vi "Outputs.vi"(8 "error in (no error)":errorcluster, 11 "State in":T1={"State"=enum."Idle", "Start Time"=timestamp(0 s since 1904-01-01), "Configuration"={"Cycle Period"=0.0, "Ismatech"={"VISA resource name"="", "Simulated?"=FALSE, "Pump Number"=1.0, "Reverse?"=FALSE}, "Masterflex"={"VISA resource name"="", "Simulated?"=FALSE, "Pump Number"=1.0, "Reverse?"=FALSE}, "Mettler"={"VISA resource name"="", "Simulated?"=FALSE}, "Bronkhorst M13 Flow Meter"={"VISA resource name"="", "Simulated?"=FALSE, "Smoothing Steps"=1}, "PID 2 Parameters"={"Input Device"=enum."Flowmeter", "Output Device"=enum."Ismatec ISM 831C", "Setpoint"=0.0, "PID gains"={"proportional gain (Kc)"=1.0, "integral time (Ti, min)"=0.01, "derivative time (Td, min)"=0.0}}, "Manual Entry"=0.0, "Auto?"=TRUE, "VICI Settings"={"VISA resource name"="", "Simulated?"=FALSE, "Pump Number"=0.0, "Reverse?"=FALSE}, "output range"={"output high"=100.0, "output low"=0.0}}, "Current Time"=timestamp(0 s since 1904-01-01), "PID 1 Parameters"={"Setpoint"=0.0, "PID gains"={"proportional gain (Kc)"=1.0, "integral time (Ti, min)"=0.01, "derivative time (Td, min)"=0.0}}, "First Iteration"=FALSE, "Data"={"Flowmeter Output"=0.0, "PID 1 Output"=0.0, "PID 2 Process Variable"=0.0, "Scale Output (g)"=0.0, "PID 2 output"=0.0, "Scale Rate of Change (g/min)"=0.0}, "Process Name"="", "Pump On?"=FALSE} {"PID 1 Parameters"."PID gains"."derivative time (Td, min)" format="%.3f"; "PID 1 Parameters"."PID gains"."integral time (Ti, min)" format="%.3f"; "PID 1 Parameters"."PID gains"."proportional gain (Kc)" format="%.3f"; "Configuration"."output range"."output low" min=0.0 max=100.0 format="%.2f"; "Configuration"."output range"."output high" format="%.2f"; "Configuration"."VICI Settings"."Pump Number" min=1.0 max=20.0 step=1.0; "Configuration"."PID 2 Parameters"."PID gains"."derivative time (Td, min)" format="%.3f"; "Configuration"."PID 2 Parameters"."PID gains"."integral time (Ti, min)" format="%.3f"; "Configuration"."PID 2 Parameters"."PID gains"."proportional gain (Kc)" format="%.3f"; "Configuration"."Bronkhorst M13 Flow Meter"."Smoothing Steps" min=1 step=1; "Configuration"."Masterflex"."Pump Number" min=1.0 max=20.0 step=1.0; "Configuration"."Ismatech"."Pump Number" min=1.0 max=20.0 step=1.0}) -> (0 "error out":errorcluster, 3 "State out":T1={"State"=enum."Idle", "Start Time"=timestamp(0 s since 1904-01-01), "Configuration"={"Cycle Period"=0.0, "Ismatech"={"VISA resource name"="", "Simulated?"=FALSE, "Pump Number"=1.0, "Reverse?"=FALSE}, "Masterflex"={"VISA resource name"="", "Simulated?"=FALSE, "Pump Number"=1.0, "Reverse?"=FALSE}, "Mettler"={"VISA resource name"="", "Simulated?"=FALSE}, "Bronkhorst M13 Flow Meter"={"VISA resource name"="", "Simulated?"=FALSE, "Smoothing Steps"=1}, "PID 2 Parameters"={"Input Device"=enum."Flowmeter", "Output Device"=enum."Ismatec ISM 831C", "Setpoint"=0.0, "PID gains"={"proportional gain (Kc)"=1.0, "integral time (Ti, min)"=0.01, "derivative time (Td, min)"=0.0}}, "Manual Entry"=0.0, "Auto?"=TRUE, "VICI Settings"={"VISA resource name"="", "Simulated?"=FALSE, "Pump Number"=0.0, "Reverse?"=FALSE}, "output range"={"output high"=100.0, "output low"=0.0}}, "Current Time"=timestamp(0 s since 1904-01-01), "PID 1 Parameters"={"Setpoint"=0.0, "PID gains"={"proportional gain (Kc)"=1.0, "integral time (Ti, min)"=0.01, "derivative time (Td, min)"=0.0}}, "First Iteration"=FALSE, "Data"={"Flowmeter Output"=0.0, "PID 1 Output"=0.0, "PID 2 Process Variable"=0.0, "Scale Output (g)"=0.0, "PID 2 output"=0.0, "Scale Rate of Change (g/min)"=0.0}, "Process Name"="", "Pump On?"=FALSE} {"PID 1 Parameters"."PID gains"."derivative time (Td, min)" format="%.3f"; "PID 1 Parameters"."PID gains"."integral time (Ti, min)" format="%.3f"; "PID 1 Parameters"."PID gains"."proportional gain (Kc)" format="%.3f"; "Configuration"."output range"."output low" min=0.0 max=100.0 format="%.2f"; "Configuration"."output range"."output high" format="%.2f"; "Configuration"."VICI Settings"."Pump Number" min=1.0 max=20.0 step=1.0; "Configuration"."PID 2 Parameters"."PID gains"."derivative time (Td, min)" format="%.3f"; "Configuration"."PID 2 Parameters"."PID gains"."integral time (Ti, min)" format="%.3f"; "Configuration"."PID 2 Parameters"."PID gains"."proportional gain (Kc)" format="%.3f"; "Configuration"."Bronkhorst M13 Flow Meter"."Smoothing Steps" min=1 step=1; "Configuration"."Masterflex"."Pump Number" min=1.0 max=20.0 step=1.0; "Configuration"."Ismatech"."Pump Number" min=1.0 max=20.0 step=1.0})   [LabVIEW 2021, in "Scale Module.lvlib" / "Scale Module Engine.lvlib"]
uses:
  Scale Module Engine.lvlib
  Ismatec ISM 831C/Ismatec ISM 831C.lvlib
  Masterflex 7550-30/Masterflex 7550-30.lvlib
  VICI M50/VICI M50.lvlib
  State Enum.ctl
  Feed Module/Controls/Scale Module Settings Cluster.ctl
  Scale Module.lvlib
  State Cluster.ctl
  Measure Instrument/PID Input Enum.ctl
  Measure Instrument/PID 2 Output Enum.ctl
  Measure Instrument/PID 2 Parameters Cluster.ctl
  Ismatec ISM 831C/Controls/Ismatech Settings Cluster.ctl
  Masterflex 7550-30/Controls/Settings Cluster.ctl
  Mettler Toledo/Controls/Settings Cluster.ctl
  Mettler Toledo/Mettler Toledo.lvlib
  Measure Instrument/PID 1 Parameters Cluster.ctl
  VICI M50/VICI Settings.ctl
  Bronkhorst M13 Flow Meter/Settings Cluster.ctl
  Bronkhorst M13 Flow Meter/Bronkhorst M13 Flow Meter.lvlib
panel:
  # "Output Instruments"
  # "Input Instruments"
  # "Output Instruments"
  # "Input Instruments"
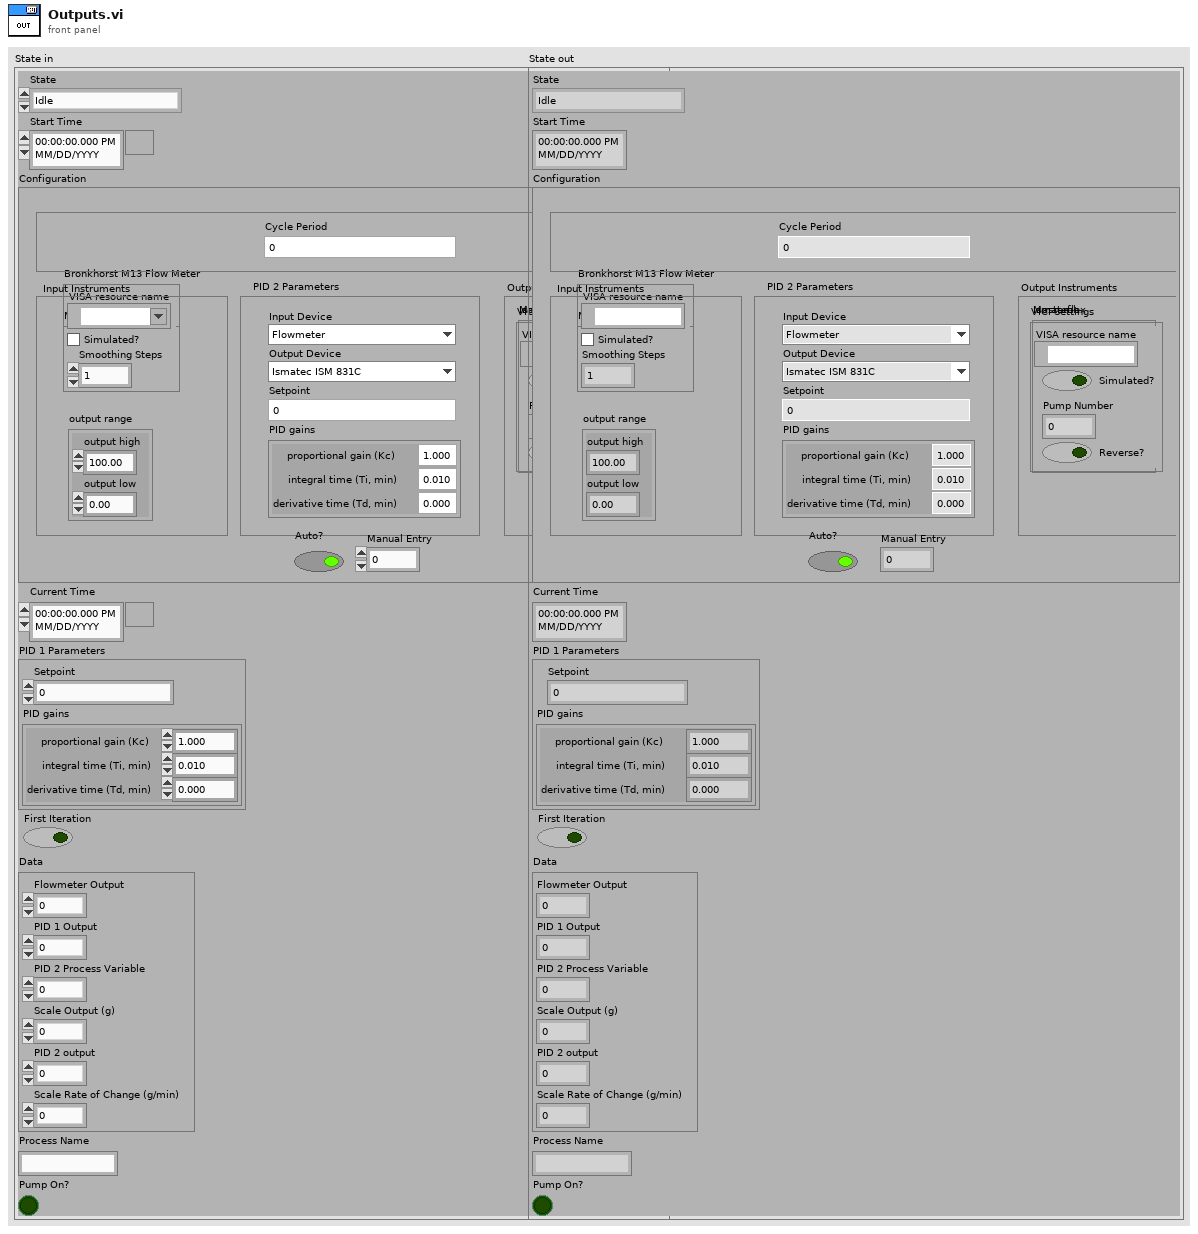
[diagram p1: front panel]
types:
  T1 = typedef "Scale Module.lvlib/Scale Module Engine.lvlib/State Cluster.ctl" = cluster{"State":T2, "Start Time":timestamp, "Configuration":T3, "Current Time":timestamp, "PID 1 Parameters":T12, "First Iteration":bool, "Data":cluster{"Flowmeter Output":dbl, "PID 1 Output":dbl, "PID 2 Process Variable":dbl, "Scale Output (g)":dbl, "PID 2 output":dbl, "Scale Rate of Change (g/min)":dbl}, "Process Name":string, "Pump On?":bool}
  T2 = typedef "Scale Module.lvlib/Scale Module Engine.lvlib/State Enum.ctl" = enum16{"Measuring", "Idle"}
  T3 = typedef "Scale Module.lvlib/Scale Module Settings Cluster.ctl" = cluster{"Cycle Period":dbl, "Ismatech":T4, "Masterflex":T5, "Mettler":T6, "Bronkhorst M13 Flow Meter":T7, "PID 2 Parameters":T8, "Manual Entry":dbl, "Auto?":bool, "VICI Settings":T11, "output range":cluster{"output high":dbl, "output low":dbl}}
  T4 = typedef "Ismatec ISM 831C.lvlib/Ismatech Settings Cluster.ctl" = cluster{"VISA resource name":refnum<visa-resource-name>, "Simulated?":bool, "Pump Number":dbl, "Reverse?":bool}
  T5 = typedef "Masterflex 7550-30.lvlib/Settings Cluster.ctl" = cluster{"VISA resource name":refnum<visa-resource-name>, "Simulated?":bool, "Pump Number":dbl, "Reverse?":bool}
  T6 = typedef "Mettler Toledo.lvlib/Settings Cluster.ctl" = cluster{"VISA resource name":refnum<visa-resource-name>, "Simulated?":bool}
  T7 = typedef "Bronkhorst M13 Flow Meter.lvlib/Settings Cluster.ctl" = cluster{"VISA resource name":refnum<visa-resource-name>, "Simulated?":bool, "Smoothing Steps":i32}
  T8 = typedef "PID 2 Parameters Cluster.ctl" = cluster{"Input Device":T9, "Output Device":T10, "Setpoint":dbl, "PID gains":cluster{"proportional gain (Kc)":dbl, "integral time (Ti, min)":dbl, "derivative time (Td, min)":dbl}}
  T9 = typedef "PID Input Enum.ctl" = enum16{"Default", "Flowmeter", "Scale Rate of Change"}
  T10 = typedef "PID 2 Output Enum.ctl" = enum16{"Default", "Ismatec ISM 4308", "Ismatec ISM 831C", "Masterflex 7550-30", "VICI M6", "VICI M50", "Tacmina QI", "KNF SIMDOS", "ASIA Type C", "FLOM UI-22-11", "SSI PR/LD", "SSI P40", "Masterflex 75211-70"}
  T11 = typedef "VICI Settings.ctl" = cluster{"VISA resource name":refnum<visa-resource-name>, "Simulated?":bool, "Pump Number":dbl, "Reverse?":bool}
  T12 = typedef "PID 1 Parameters Cluster.ctl" = cluster{"Setpoint":dbl, "PID gains":cluster{"proportional gain (Kc)":dbl, "integral time (Ti, min)":dbl, "derivative time (Td, min)":dbl}}
  T13 = typedef "Ismatec ISM 831C.lvlib/Ismatech ISM831C Settings Cluster.ctl" = cluster{"VISA resource name":refnum<visa-resource-name>, "Simulated?":bool, "Pump Number":dbl, "Reverse?":bool}
  T14 = typedef "Settings Cluster.ctl" = cluster{"VISA resource name":refnum<visa-resource-name>, "Simulated?":bool, "Pump Number":dbl, "Reverse?":bool}
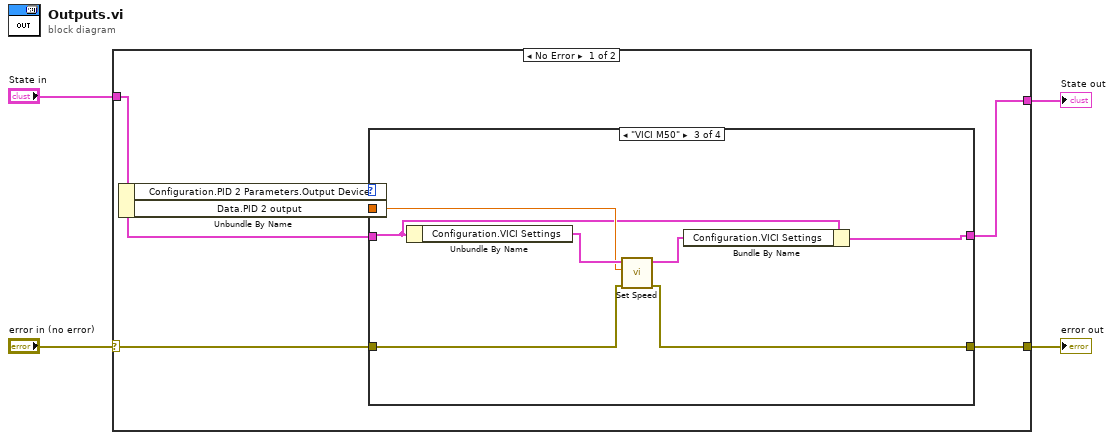
[diagram p0: block diagram]
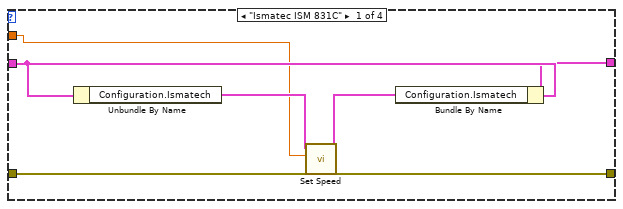
[diagram p2: hidden frame]
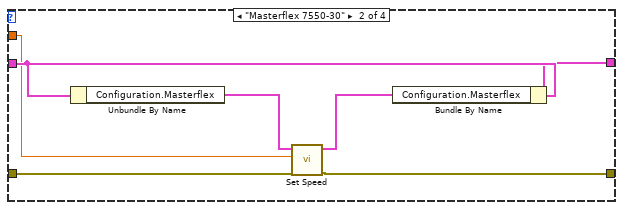
[diagram p3: hidden frame]
diagram:
  n1 = case shown="No Error" "error in (no error)" {
    selector: "error in (no error)" -> [w8 w35]
    tunnel: [w7 w35] -> w3
    tunnel: "State in" -> [w5 w34]
    tunnel: [w6 w34] -> w1
    frame No Error {
      n2 = Unbundle By Name(w5) -> ("Configuration.PID 2 Parameters.Output Device"=w10:T10, "Data.PID 2 output"=w9:dbl)
      n3 = case shown="\"VICI M50\"" w10 {
        tunnel: w9 -> [w11 w18 w30 _]
        tunnel: w8 -> [w17 w20 w29 w32]
        tunnel: [w16 w19 w28 w32] -> w7
        tunnel: w5 -> [w15 w24 w25 w33]
        tunnel: [w12 w23 w27 w33] -> w6
        frame "Ismatec ISM 831C" {
          n4 = Unbundle By Name(w15) -> ("Configuration.Ismatech"=w14:T4)
          n5 = call "Set Speed.vi"("error in (no error)"=w17, "Speed (%)"=w11, "Ismatech Settings In"=w14) -> ("error out"=w16:errorcluster, "Ismatech Settings Out"=w13:T13)  [unwired: 6 in, 1 out]
          n6 = Bundle By Name(cluster=w15, "Configuration.Ismatech"=w13) -> (w12:T1)
        }
        frame "Masterflex 7550-30" {
          n7 = Unbundle By Name(w24) -> ("Configuration.Masterflex"=w22:T5)
          n8 = call "Set Speed.vi"("error in (no error)"=w20, "speed"=w18, "Masterflex Settings in"=w22) -> ("error out"=w19:errorcluster, "Masterflex Settings out"=w21:T5)  [unwired: 6 in, 1 out]
          n9 = Bundle By Name(cluster=w24, "Configuration.Masterflex"=w21) -> (w23:T1)
        }
        frame "VICI M50" {
          n10 = Unbundle By Name(w25) -> ("Configuration.VICI Settings"=w31:T11)
          n11 = call "Set Speed.vi"("error in (no error)"=w29, "speed"=w30, "VICI Settings In"=w31) -> ("error out"=w28:errorcluster, "VICI Settings Out"=w26:T14)  [unwired: 6 in, 1 out]
          n12 = Bundle By Name(cluster=w25, "Configuration.VICI Settings"=w26) -> (w27:T1)
        }
        frame "Default", Default {
        }
      }
    }
    frame Error {
    }
  }
  "error out" <- w3
  "State out" <- w1
